vi "Post - NT Enum (Index & Choices).vi"(6 "timestamp":timestamp, 7 "PV name":string, 8 "error in (no error)":errorcluster, 9 "choices":string[](array[string]), 10 "index":u16, 11 "Server in":refnum<class "Server.lvclass">) -> (0 "error out":errorcluster, 3 "Server out":refnum<class "Server.lvclass">)   [LabVIEW 2020, in "PV Access.lvlib" / "PVA Server.lvlib" / "Server.lvclass"]
doc: "If you just want to set the index, leave the <B>choices in</B> control unset. Only array containg at least one element will be used."
uses:
  Server.lvclass
  Server.lvclass/Server.ctl
  PV Data/PV Data/PV Data.lvclass
  Source/Source.lvclass
  PV Data/PV Data/Write Field - I32.vi
  PV Data/PV Data/Write Field - String Array.vi
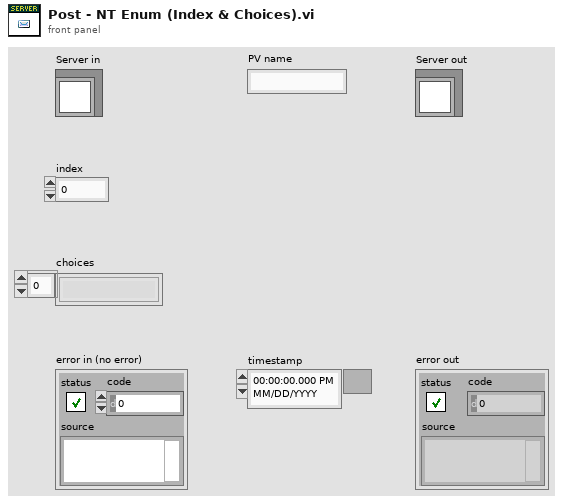
[diagram p1: front panel]
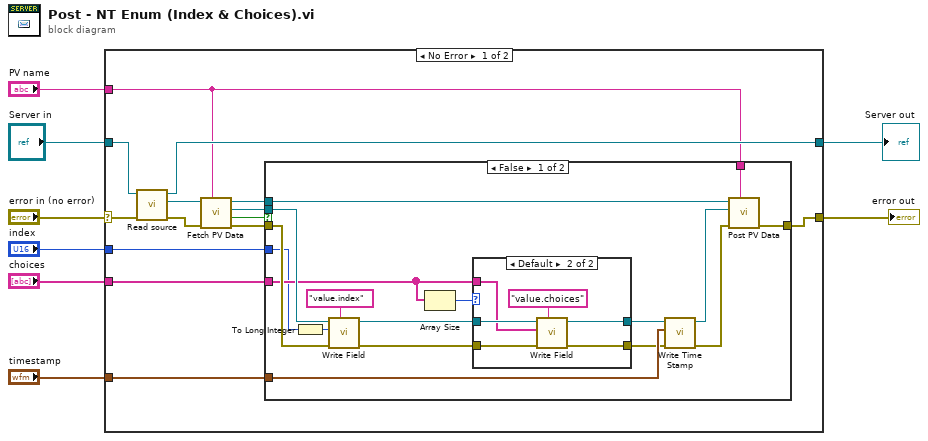
[diagram p0: block diagram]
diagram:
  n1 = case shown="No Error" "error in (no error)" {
    selector: "error in (no error)" -> [w20 w50]
    tunnel: [w13 w50] -> w3
    tunnel: [w21 w49] -> w2
    tunnel: "Server in" -> [w22 w49]
    tunnel: "PV name" -> [w14 _]
    tunnel: "index" -> [w12 _]
    tunnel: "timestamp" -> [w16 _]
    tunnel: "choices" -> [w11 _]
    frame No Error {
      n2 = call "Read source.vi"("error in (no error)"=w20, "Server in"=w22) -> ("error out"=w18:errorcluster, "Source"=w19:refnum<class "Source.lvclass">, "Server out"=w21:refnum<class "Server.lvclass">)  [unwired: 7 in]
      n3 = call "Fetch PV Data.vi"("PV name"=w14, "error in"=w18, "Source in"=w19) -> ("error out"=w9:errorcluster, "PV not found?"=w10:bool, "PV Data out"=w17:refnum<class "PV Data.lvclass">, "Source out"=w15:refnum<class "Source.lvclass">)  [unwired: 5 in]
      n4 = case shown="False" w10 {
        tunnel: w12 -> [w24 _]
        tunnel: w17 -> [w39 _]
        tunnel: w9 -> [w38 w48]
        tunnel: w16 -> [w36 _]
        tunnel: w15 -> [w33 _]
        tunnel: w14 -> [w32 _]
        tunnel: [w31 w48] -> w13
        tunnel: w11 -> [w25 _]
        frame False {
          n5 = To Long Integer(number=w24) -> (32bit integer=w23:i32)
          n6 = call-poly "Write Field.vi"("field name"="value.index", "error in"=w38, "value"=w23, "PV Data in"=w39) -> ("error out"=w29:errorcluster, "PV Data out"=w30:refnum<class "PV Data.lvclass">)  [unwired: 5 in, 1 out]
          n7 = Array Size(array=w25) -> (size(s)=w26:i32)
          n8 = case shown="Default" w26 {
            tunnel: w30 -> [w41 w46]
            tunnel: w29 -> [w40 w45]
            tunnel: [w40 w44] -> w28
            tunnel: [w41 w43] -> w27
            tunnel: w25 -> [_ w42]
            frame 0 {
            }
            frame Default {
              n9 = call-poly "Write Field.vi"("field name"="value.choices", "error in"=w45, "value"=w42, "PV Data in"=w46) -> ("error out"=w44:errorcluster, "PV Data out"=w43:refnum<class "PV Data.lvclass">)  [unwired: 5 in, 1 out]
            }
          }
          n10 = call "Write Time Stamp.vi"("error in"=w28, "timestamp in"=w36, "PV Data in"=w27) -> ("error out"=w35:errorcluster, "PV Data out"=w34:refnum<class "PV Data.lvclass">)  [unwired: 5 in, 2 out]
          n11 = call "Post PV Data.vi"("PV name"=w32, "error in"=w35, "PV Data in"=w34, "Source in"=w33) -> ("error out"=w31:errorcluster)  [unwired: 6 in, 1 out]
        }
        frame True {
        }
      }
    }
    frame Error {
    }
  }
  "error out" <- w3
  "Server out" <- w2
